vi "sub_identity-matrix.vi"(11 "STATE_SIZE":i32) -> (3 "identity":dbl[][](array[numeric]))   [LabVIEW 2019]
uses:
  <vilib>/Analysis/Matrix/Datatypes/RealMatrix.ctl
  <vilib>/Analysis/Matrix/Numeric/Conversions/Array To Matrix - RA2.vi
  <vilib>/Analysis/Matrix/NI_Matrix.lvlib
panel:
  out "Real Matrix":T1 caption="실수 행렬"
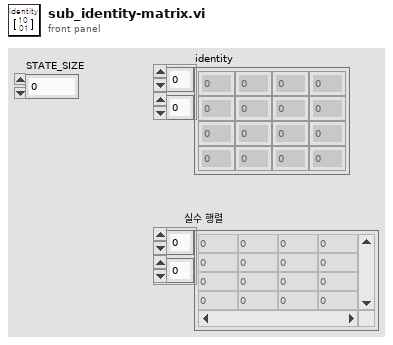
[diagram p1: front panel]
types:
  T1 = typedef "NI_Matrix.lvlib/RealMatrix.ctl" = dbl[][]
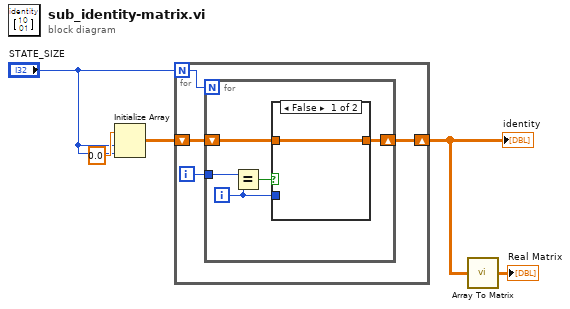
[diagram p0: block diagram]
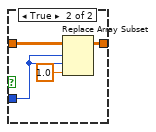
[diagram p2: hidden frame]
diagram:
  n1 = Initialize Array(0.0 ("원소"), "STATE_SIZE", "STATE_SIZE") -> (w5:dbl[][])
  n2 = for {
    N: "STATE_SIZE" -> [w9]
    shift-right: [w6] -> w2
    shift-left: w5 -> [w7]
    i -> [w8]
    n3 = for {
      N: w9 -> [_]
      tunnel: w8 -> [w14]
      shift-right: [w12] -> w6
      shift-left: w7 -> [w13]
      i -> [w11]
      n4 = Equal?(x=w14, y=w11) -> (x = y?=w10:bool)
      n5 = case shown="False" w10 {
        tunnel: w13 -> [w15 w19]
        tunnel: [w15 w18] -> w12
        tunnel: w11 -> [_ w17]
        frame False {
        }
        frame True {
          n6 = Replace Array Subset(array=w19, new element=1.0 ("새 원소/부분배열"), index (row)=w17, index (col)=w17) -> (w18:dbl[][])
        }
      }
    }
  }
  "identity" <- w2
  n7 = call-poly <vilib>:"Array To Matrix.vi"("Real 2D Array"=w2) -> ("Real Matrix"=→"Real Matrix":T1)
